vi "ModuFPGA.vi"() -> ()   [LabVIEW 2012]
uses:
  <vilib>/Platform/TimedLoop/XDataNode/timing_clust.ctl
  <vilib>/Platform/TimedLoop/XDataNode/nitl_modes.ctl
  <vilib>/Platform/TimedLoop/XDataNode/wakeup.ctl
  <vilib>/rvi/DataTransferAndStorage/Container/Common/niFpgaContainerMetaDataKey.ctl
  <vilib>/rvi/DataTransferAndStorage/Container/Common/niFpgaContainerState.ctl
  <vilib>/rvi/DataTransferAndStorage/Container/Common/niFpgaDataTypeControl.ctl
  <vilib>/rvi/DataTransferAndStorage/Container/Common/niFpgaContainerImplementationControl.ctl
  <vilib>/rvi/DataTransferAndStorage/Container/Common/niFpgaContainerArbitrationOptionsControl.ctl
  <vilib>/rvi/DataTransferAndStorage/Container/Common/niFpgaTransferTypeControl.ctl
  <vilib>/rvi/DataTransferAndStorage/Container/Common/niFpgaContainerInitializationParameters.ctl
  <vilib>/rvi/Memory/Memory_Types/niFpgaMemoryInterfaceConfiguration.ctl
  <vilib>/rvi/FIFO/Fifo_Types/niFpgaFifoControlLogicControl.ctl
  <vilib>/rvi/eio/common/nirviEmuTemplateMethod_errors.vi
  <vilib>/rvi/FIFO/Fifo_Resource/nirvififoEmulationSetSize.vi
  <vilib>/rvi/DataTransferAndStorage/Container/Common/niFpgaContainerGetUniqueNameForEmu.vi
  <vilib>/rvi/Emulation/niFpgaSctlEmulationRegisterWithScheduler.vi
  <vilib>/rvi/Emulation/niFpgaSctlEmulationScheduler.vi
  <vilib>/rvi/DataTransferAndStorage/Container/Common/niFpgaContainerSetEmuInfo.vi
  <vilib>/rvi/eio/common/nirviEmuReportErrorAndStop.vi
  <vilib>/rvi/Emulation/niFpgaSctlEmulationFifoFullMgr.vi
  <vilib>/rvi/errors/niFpgaSetErrorForExecOnDevCompSimple.vi
  <vilib>/rvi/Memory/Memory_Emulation/niFpgaMemoryEmulationCacheClearOnFirstRun.vi
  <vilib>/rvi/Memory/Memory_Emulation/nirvimemoryEmulationManagerCache_MakeExclusive.vi
  <vilib>/rvi/Memory/Memory_Emulation/niFpgaMemoryEmulationValidateCache.vi
  <vilib>/rvi/Memory/Memory_Emulation/nirvimemoryEmulationManagerCache_ReleaseExclusive.vi
  <vilib>/rvi/Memory/Memory_Emulation/nirvimemoryEmulationManagerCache_InsertValue.vi
  <vilib>/Utility/error.llb/Clear Errors.vi
  <vilib>/rvi/Memory/Memory_Emulation/nirvimemoryEmulationManagerCache_GetValue.vi
  <vilib>/rvi/Emulation/niFpgaSctlEmulationResourceMgr.vi
  <vilib>/eio/EIONode/EIONode.xnode
  <vilib>/Platform/TimedLoop/XDataNode/XDataNode.xnode
  <vilib>/rvi/DataTransferAndStorage/Container/XNode/niFpgaContainer.xnode
  <vilib>/rvi/FIFO/Fifo_Resource/nirvififoEmulationClear.vi
  <vilib>/rvi/LocalResourceManager/LocalResourceManager.xnode
  <vilib>/rvi/FIFO/Fifo_Resource/nirvififoEmulationRead.vi
  <vilib>/rvi/Memory/Memory_Emulation/nirvimemoryEmulation.vi
  <vilib>/rvi/FIFO/Fifo_Resource/nirvififoEmulationWrite.vi
  <vilib>/Platform/TimedLoop/XDataNode/XDNodeRunTimeDep.lvlib
panel:
  out "Total number of pulses sent ch 0":u64
  out "Total number of pulses sent ch 1":u64
  out "Total number of pulses sent ch 2":u64
  out "Total number of pulses sent ch 3":u64
  out "Total number of pulses sent ch 4":u64
  out "Total number of pulses sent ch 5":u64
  out "Total number of pulses sent ch 6":u64
  out "Total number of pulses sent ch 7":u64
  out "IO Module\\ADC Error A":bool
  out "IO Module\\ADC Error B":bool
  out "IO Module\\Pll Unlocked":bool
  in  "Record Size only data":u32=95
  out "DMA FIFO Timed Out?":bool
  in  "circular buffer length":u32=1000
  in  "location":i16(ring) items=["Purdue", "NIKHEF", "Zurich", "???"]
  in  "Trigger 0":i16=4000
  in  "Trigger 1":i16=4000
  in  "Trigger 2":i16=4000
  in  "Trigger 3":i16=4000
  in  "Trigger 4":i16=4000
  in  "Trigger 5":i16=4000
  in  "Trigger 6":i16=4000
  in  "Trigger 7":i16=4000
  in  "# of pretrigger":u32=20
  in  "initial value":u64
  in  "channel 0 on/off":bool
  in  "channel 2 on/off":bool
  in  "channel 1 on/off":bool
  in  "channel 3 on/off":bool
  in  "channel 4 on/off":bool
  in  "channel 5 on/off":bool
  in  "channel 6 on/off":bool
  in  "channel 7 on/off":bool
  in  "Testpulse duration (20 ns ticks)":u32=1
  in  "Testpulse Separation (20 ns ticks)":u32=500
  in  "Testpulse Time Delay (20 ns ticks)":u32=15
  in  "Testpulser On/Off":bool
  out "Init Done":bool
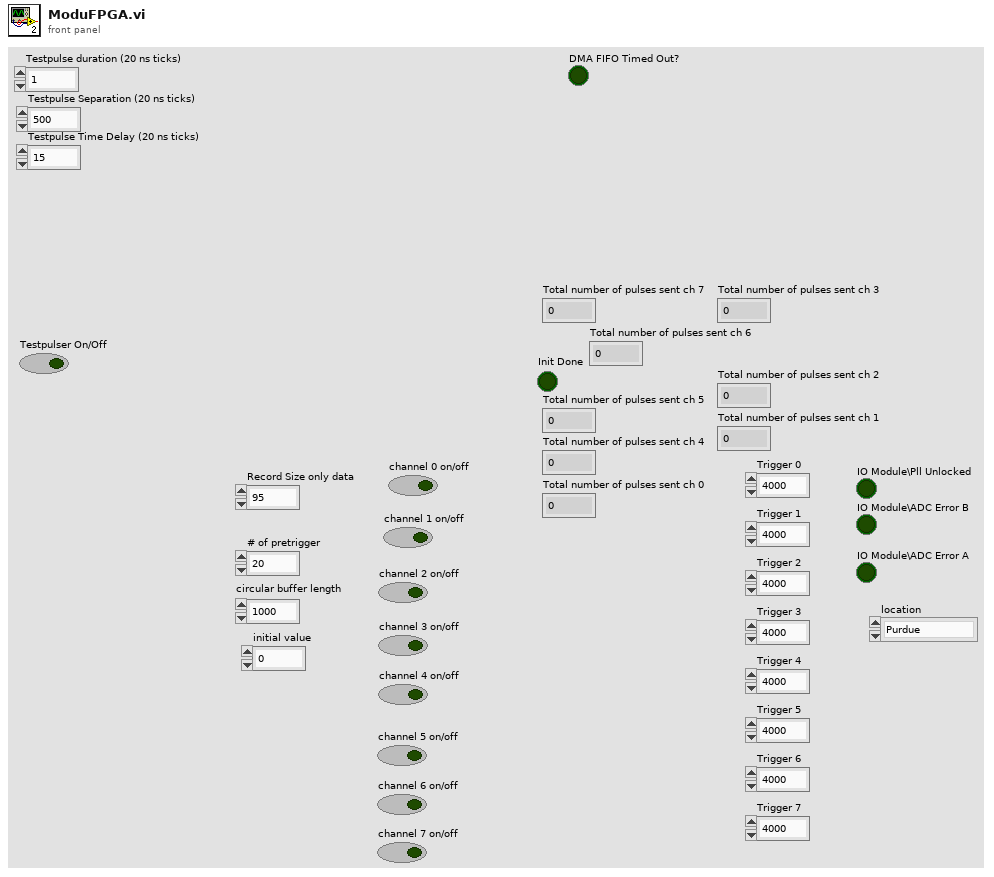
[diagram p1: front panel]
types:
  T1 = typedef "XDNodeRunTimeDep.lvlib/timing_clust.ctl" = cluster{"Expected End [f-1]":u64, "Actual End [f-1]":u64, "Finished Late? [f-1]":bool, "Expected End [i-1]":u64, "Actual End [i-1]":u64, "Finished Late? [i-1]":bool, "Expected Start [i]":u64, "Actual Start [i]":u64, "Expected Start [f]":u64, "Actual Start [f]":u64, "Source Name":string, "Structure Name":string, "Period":i64, "Deadline":i64, "Offset":i64, "Start":i64, "Priority":i32, "Timeout":i32, "Mode":T2, "Wakeup Reason":T3, "Error":errorcluster, "Source Type":string, "Secondary Source Type":string, "Global End Time":u64, "Global Start Time":u64, "Frame Duration":u64, "Iteration Duration":u64, "Assigned CPU":i32, "I/O Scan Engine Mode":u32}
  T2 = typedef "XDNodeRunTimeDep.lvlib/nitl_modes.ctl" = enum32{"No Change", "Process missed periods, maintain original phase", "Discard missed periods, maintain original phase", "Process missed periods, ignore original phase", "Discard missed periods, ignore original phase"}
  T3 = typedef "XDNodeRunTimeDep.lvlib/wakeup.ctl" = enum32{"Normal", "Aborted", "Asynchronous wakeup", "Timing source error", "Timed loop error", "Timeout"}
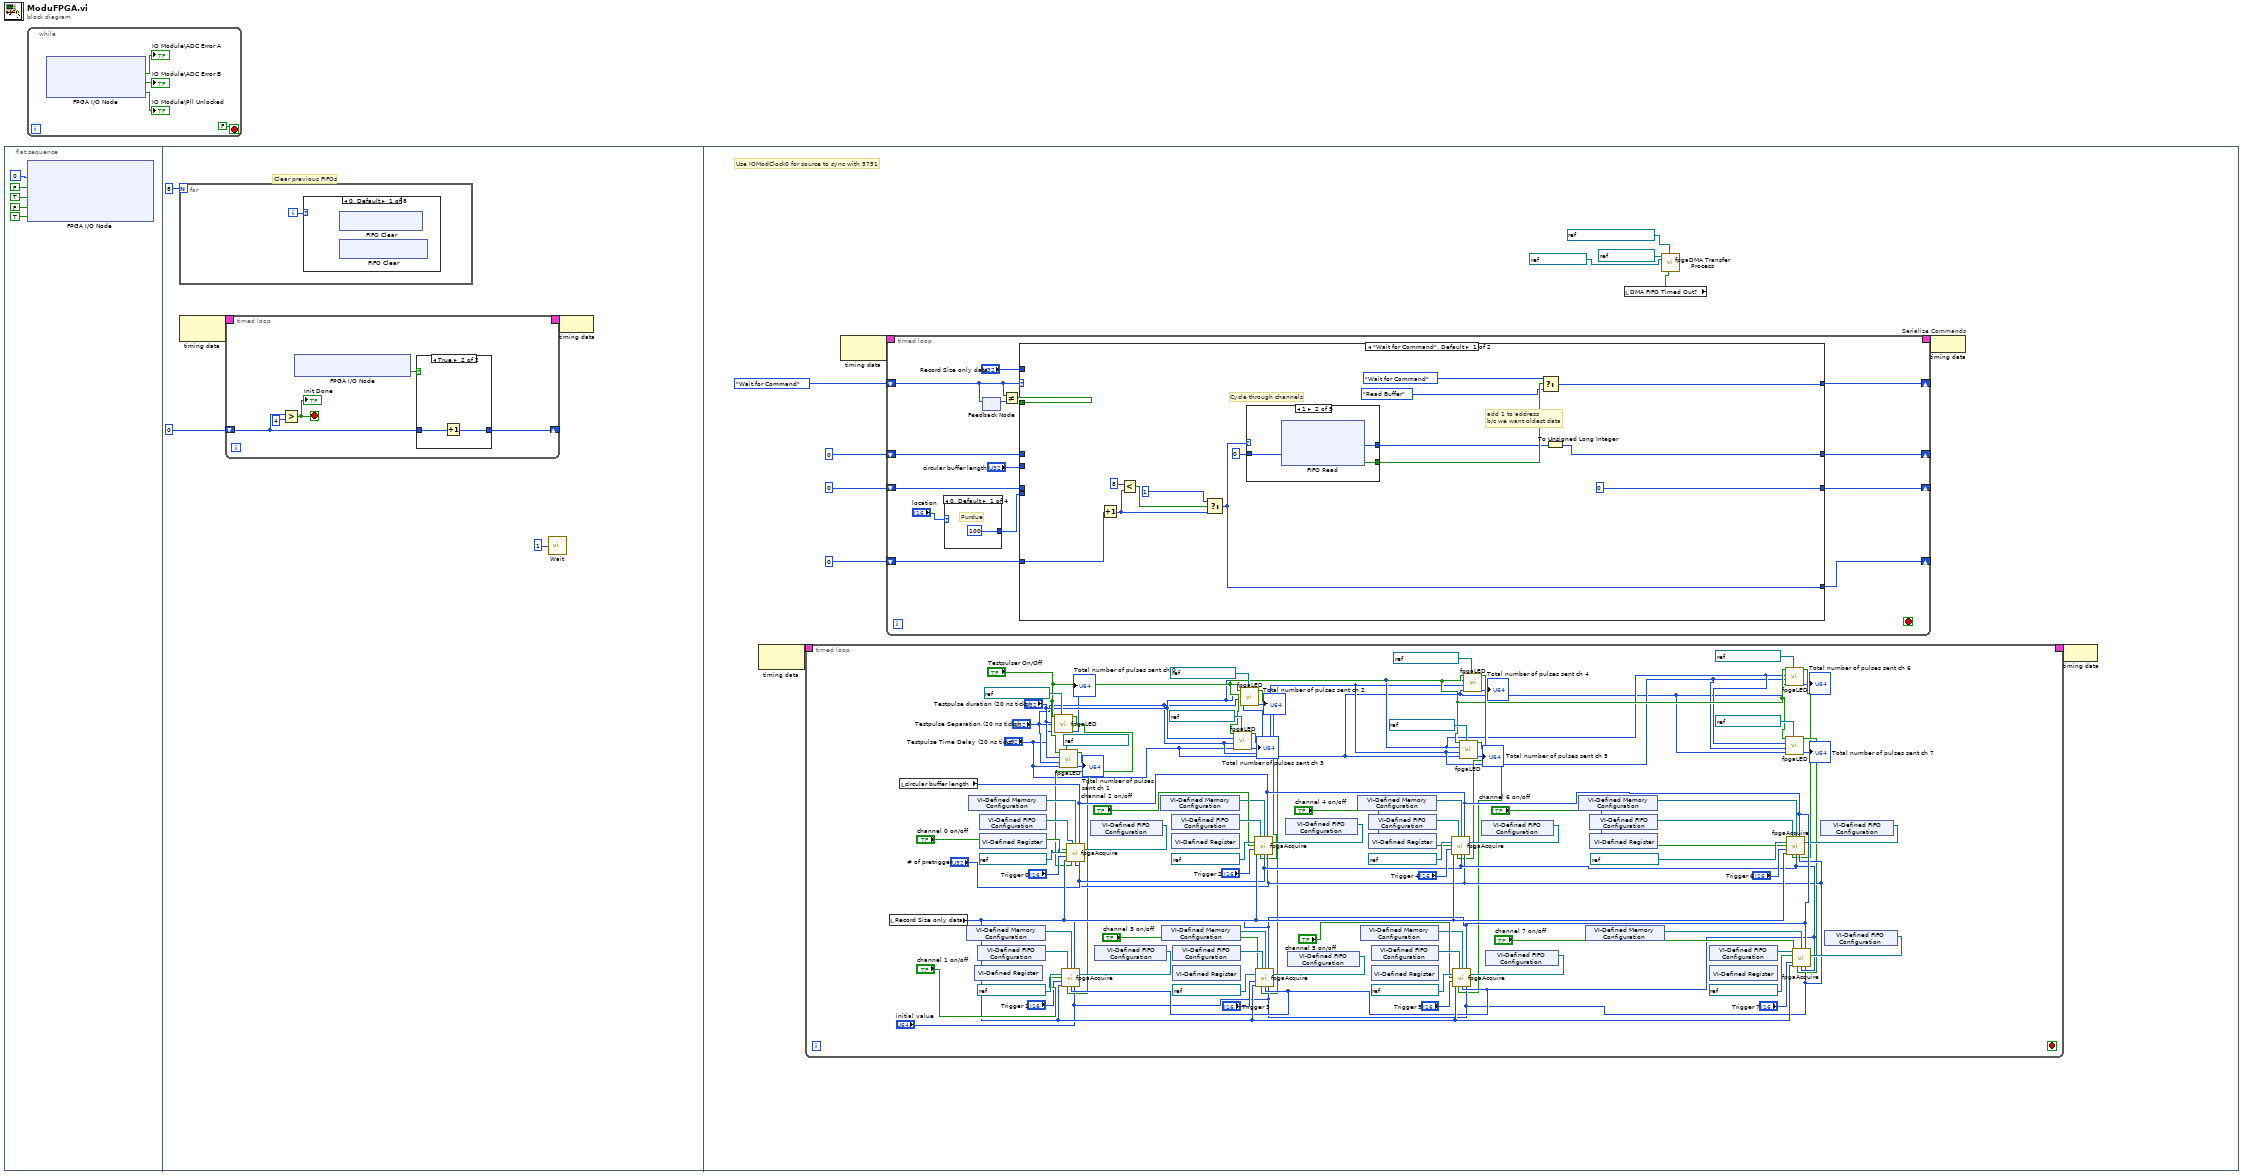
[diagram p0: block diagram]
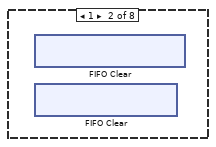
[diagram p2: hidden frame]
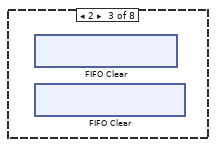
[diagram p3: hidden frame]
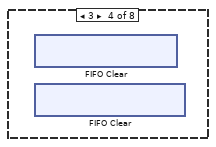
[diagram p4: hidden frame]
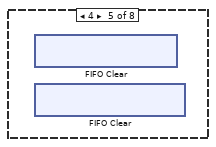
[diagram p5: hidden frame]
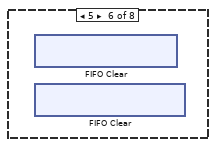
[diagram p6: hidden frame]
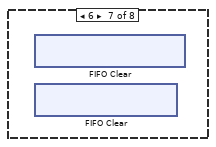
[diagram p7: hidden frame]
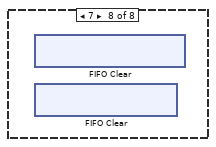
[diagram p8: hidden frame]
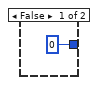
[diagram p9: hidden frame]
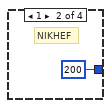
[diagram p10: hidden frame]
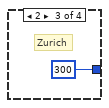
[diagram p11: hidden frame]
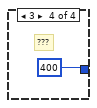
[diagram p12: hidden frame]
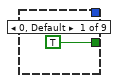
[diagram p13: hidden frame]
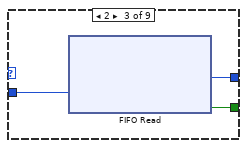
[diagram p14: hidden frame]
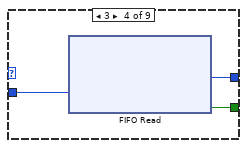
[diagram p15: hidden frame]
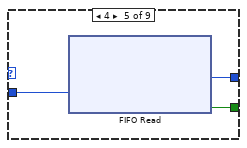
[diagram p16: hidden frame]
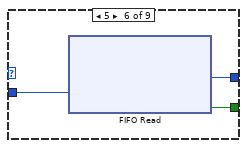
[diagram p17: hidden frame]
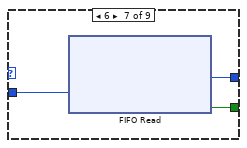
[diagram p18: hidden frame]
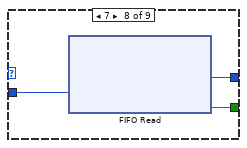
[diagram p19: hidden frame]
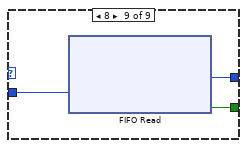
[diagram p20: hidden frame]
diagram:
  n1 = flat-sequence {
    frame #0 {
      n2 = xnode "FPGA I/O Node"("IO Module\\Sample Clock Select"=u8 0 ("IO Module\\Sample Clock Select"), "IO Module\\Force Initialization"=FALSE ("IO Module\\Force Initialization"), "IO Module\\Force Initialization"=TRUE ("IO Module\\Force Initialization"), "IO Module\\Force Initialization"=FALSE ("IO Module\\Force Initialization"), "IO Module\\Digital Output Enable"=TRUE ("IO Module\\Digital Output Enable")) -> ()  [unwired: 5 in, 5 out]
    }
    frame #1 {
      # "Clear previous FIFOs"
      n3 = for {
        N: 8 -> [_]
        i -> [w11]
        n4 = case shown="0, Default" w11 {
          frame 0, Default {
            n5 = xnode ("FIFO Clear")() -> ()  [unwired: 1 in, 1 out]
            n6 = xnode ("FIFO Clear")() -> ()  [unwired: 1 in, 1 out]
          }
          frame 1 {
            n7 = xnode ("FIFO Clear")() -> ()  [unwired: 1 in, 1 out]
            n8 = xnode ("FIFO Clear")() -> ()  [unwired: 1 in, 1 out]
          }
          frame 2 {
            n9 = xnode ("FIFO Clear")() -> ()  [unwired: 1 in, 1 out]
            n10 = xnode ("FIFO Clear")() -> ()  [unwired: 1 in, 1 out]
          }
          frame 3 {
            n11 = xnode ("FIFO Clear")() -> ()  [unwired: 1 in, 1 out]
            n12 = xnode ("FIFO Clear")() -> ()  [unwired: 1 in, 1 out]
          }
          frame 4 {
            n13 = xnode ("FIFO Clear")() -> ()  [unwired: 1 in, 1 out]
            n14 = xnode ("FIFO Clear")() -> ()  [unwired: 1 in, 1 out]
          }
          frame 5 {
            n15 = xnode ("FIFO Clear")() -> ()  [unwired: 1 in, 1 out]
            n16 = xnode ("FIFO Clear")() -> ()  [unwired: 1 in, 1 out]
          }
          frame 6 {
            n17 = xnode ("FIFO Clear")() -> ()  [unwired: 1 in, 1 out]
            n18 = xnode ("FIFO Clear")() -> ()  [unwired: 1 in, 1 out]
          }
          frame 7 {
            n19 = xnode ("FIFO Clear")() -> ()  [unwired: 1 in, 1 out]
            n20 = xnode ("FIFO Clear")() -> ()  [unwired: 1 in, 1 out]
          }
        }
      }
      n21 = node-c288() -> (w10:T1)  [unwired: 1 in]
      n22 = timed-loop {
        shift-right: [w15] -> _
        shift-left: u16 0 -> [w14]
        timing: w10 -> [_]
        timing-out: [_] -> w9
        stop <- w12 stop-if-true
        n23 = Greater?(x=w14, y=u16 4) -> (0:w12:bool)
        "Init Done" <- w12
        n24 = xnode "FPGA I/O Node"() -> ("IO Module\\Initialization Done"=w16:bool)  [unwired: 1 in, 1 out]
        n25 = case shown="True" w16 {
          tunnel: [u16 0 w19] -> w15
          tunnel: w14 -> [_ w18]
          frame False {
          }
          frame True {
            n26 = Increment(x=w18) -> (x+1=w19:u16)
          }
        }
      }
      n27 = call "Wait"("Count(mSec)"=u32 1) -> ()  [unwired: 1 out]
      n28 = node-c288(w9) -> ()
    }
    frame #2 {
      # "Use IOModClock0 for source to sync with 5751"
      n29 = node-c288() -> (w29:T1)  [unwired: 1 in]
      n30 = timed-loop {
        timing: w29 -> [_]
        timing-out: [_] -> w28
        stop <- _ stop-if-true
        n31 = local read "Record Size only data"() -> (w91:u32)
        n32 = local read "circular buffer length"() -> (w66:u32)
        n33 = xnode "VI-Defined Memory Configuration"() -> ("Memory Out"=w67:refnum<k21>)
        n34 = xnode "VI-Defined Memory Configuration"() -> ("Memory Out"=w74:refnum<k21>)
        n35 = xnode "VI-Defined Register"() -> ()  [unwired: 1 out]
        n36 = xnode "VI-Defined FIFO Configuration"() -> ("FIFO Out"=w115:refnum<k21>)
        n37 = xnode "VI-Defined FIFO Configuration"() -> ("FIFO Out"=w92:refnum<k21>)
        n38 = xnode "VI-Defined Register"() -> ()  [unwired: 1 out]
        n39 = call "fpgaLED.vi"("FPGA I/O In"=refnum<k21> "IO Module\\D0 0", "Testpulse Time Delay (20 ns ticks)"="Testpulse Time Delay (20 ns ticks)", "Testpulse Separation (20 ns ticks)"="Testpulse Separation (20 ns ticks)", "Testpulse duration (20 ns ticks)"="Testpulse duration (20 ns ticks)", "Testpulser On/Off"="Testpulser On/Off") -> ("Total number of pulses sent"=→"Total number of pulses sent ch 0":u64, "Is Test Pulse?"=w48:bool)  [unwired: 5 in]
        n40 = call "fpgaLED.vi"("FPGA I/O In"=refnum<k21> "IO Module\\D0 1", "Testpulse Time Delay (20 ns ticks)"="Testpulse Time Delay (20 ns ticks)", "Testpulse Separation (20 ns ticks)"="Testpulse Separation (20 ns ticks)", "Testpulse duration (20 ns ticks)"="Testpulse duration (20 ns ticks)", "Testpulser On/Off"="Testpulser On/Off") -> ("Total number of pulses sent"=→"Total number of pulses sent ch 1":u64, "Is Test Pulse?"=w49:bool)  [unwired: 5 in]
        n41 = xnode "VI-Defined FIFO Configuration"() -> ("FIFO Out"=w64:refnum<k21>)
        n42 = call "fpgaAcquire.vi"("Command FIFO"=w92, "Circular Buffer Mem"=w74, "circular buffer length"=w66, "FPGA I/O In"=refnum<k21> "IO Module\\AI A0", "Timing FIFO"=w64, "channel on/off"="channel 0 on/off", "Trigger"="Trigger 0", "Samples to Acquire"=w91, "Is Test Pulse?"=w48, "# of pretrigger"="# of pretrigger", "timing"="initial value") -> ()  [unwired: 5 in]
        n43 = xnode "VI-Defined FIFO Configuration"() -> ("FIFO Out"=w65:refnum<k21>)
        n44 = call "fpgaAcquire.vi"("Command FIFO"=w115, "Circular Buffer Mem"=w67, "circular buffer length"=w66, "FPGA I/O In"=refnum<k21> "IO Module\\AI A1", "Timing FIFO"=w65, "channel on/off"="channel 1 on/off", "Trigger"="Trigger 1", "Samples to Acquire"=w91, "Is Test Pulse?"=w49, "# of pretrigger"="# of pretrigger", "timing"="initial value") -> ()  [unwired: 5 in]
        n45 = xnode "VI-Defined Memory Configuration"() -> ("Memory Out"=w73:refnum<k21>)
        n46 = xnode "VI-Defined Memory Configuration"() -> ("Memory Out"=w68:refnum<k21>)
        n47 = xnode "VI-Defined FIFO Configuration"() -> ("FIFO Out"=w113:refnum<k21>)
        n48 = xnode "VI-Defined Register"() -> ()  [unwired: 1 out]
        n49 = xnode "VI-Defined FIFO Configuration"() -> ("FIFO Out"=w114:refnum<k21>)
        n50 = xnode "VI-Defined Register"() -> ()  [unwired: 1 out]
        n51 = call "fpgaLED.vi"("FPGA I/O In"=refnum<k21> "IO Module\\D0 3", "Testpulse Time Delay (20 ns ticks)"="Testpulse Time Delay (20 ns ticks)", "Testpulse Separation (20 ns ticks)"="Testpulse Separation (20 ns ticks)", "Testpulse duration (20 ns ticks)"="Testpulse duration (20 ns ticks)", "Testpulser On/Off"="Testpulser On/Off") -> ("Total number of pulses sent"=→"Total number of pulses sent ch 3":u64, "Is Test Pulse?"=w51:bool)  [unwired: 5 in]
        n52 = call "fpgaLED.vi"("FPGA I/O In"=refnum<k21> "IO Module\\D0 2", "Testpulse Time Delay (20 ns ticks)"="Testpulse Time Delay (20 ns ticks)", "Testpulse Separation (20 ns ticks)"="Testpulse Separation (20 ns ticks)", "Testpulse duration (20 ns ticks)"="Testpulse duration (20 ns ticks)", "Testpulser On/Off"="Testpulser On/Off") -> ("Total number of pulses sent"=→"Total number of pulses sent ch 2":u64, "Is Test Pulse?"=w50:bool)  [unwired: 5 in]
        n53 = xnode "VI-Defined FIFO Configuration"() -> ("FIFO Out"=w63:refnum<k21>)
        n54 = call "fpgaAcquire.vi"("Command FIFO"=w113, "Circular Buffer Mem"=w73, "circular buffer length"=w66, "FPGA I/O In"=refnum<k21> "IO Module\\AI A2", "Timing FIFO"=w63, "channel on/off"="channel 2 on/off", "Trigger"="Trigger 2", "Samples to Acquire"=w91, "Is Test Pulse?"=w50, "# of pretrigger"="# of pretrigger", "timing"="initial value") -> ()  [unwired: 5 in]
        n55 = xnode "VI-Defined FIFO Configuration"() -> ("FIFO Out"=w62:refnum<k21>)
        n56 = call "fpgaAcquire.vi"("Command FIFO"=w114, "Circular Buffer Mem"=w68, "circular buffer length"=w66, "FPGA I/O In"=refnum<k21> "IO Module\\AI A3", "Timing FIFO"=w62, "channel on/off"="channel 3 on/off", "Trigger"="Trigger 3", "Samples to Acquire"=w91, "Is Test Pulse?"=w51, "# of pretrigger"="# of pretrigger", "timing"="initial value") -> ()  [unwired: 5 in]
        n57 = xnode "VI-Defined Memory Configuration"() -> ("Memory Out"=w72:refnum<k21>)
        n58 = xnode "VI-Defined Memory Configuration"() -> ("Memory Out"=w69:refnum<k21>)
        n59 = xnode "VI-Defined Register"() -> ()  [unwired: 1 out]
        n60 = xnode "VI-Defined FIFO Configuration"() -> ("FIFO Out"=w109:refnum<k21>)
        n61 = xnode "VI-Defined FIFO Configuration"() -> ("FIFO Out"=w110:refnum<k21>)
        n62 = xnode "VI-Defined Register"() -> ()  [unwired: 1 out]
        n63 = call "fpgaLED.vi"("FPGA I/O In"=refnum<k21> "IO Module\\D0 5", "Testpulse Time Delay (20 ns ticks)"="Testpulse Time Delay (20 ns ticks)", "Testpulse Separation (20 ns ticks)"="Testpulse Separation (20 ns ticks)", "Testpulse duration (20 ns ticks)"="Testpulse duration (20 ns ticks)", "Testpulser On/Off"="Testpulser On/Off") -> ("Total number of pulses sent"=→"Total number of pulses sent ch 5":u64, "Is Test Pulse?"=w53:bool)  [unwired: 5 in]
        n64 = call "fpgaLED.vi"("FPGA I/O In"=refnum<k21> "IO Module\\D0 4", "Testpulse Time Delay (20 ns ticks)"="Testpulse Time Delay (20 ns ticks)", "Testpulse Separation (20 ns ticks)"="Testpulse Separation (20 ns ticks)", "Testpulse duration (20 ns ticks)"="Testpulse duration (20 ns ticks)", "Testpulser On/Off"="Testpulser On/Off") -> ("Total number of pulses sent"=→"Total number of pulses sent ch 4":u64, "Is Test Pulse?"=w52:bool)  [unwired: 5 in]
        n65 = xnode "VI-Defined FIFO Configuration"() -> ("FIFO Out"=w58:refnum<k21>)
        n66 = call "fpgaAcquire.vi"("Command FIFO"=w109, "Circular Buffer Mem"=w72, "circular buffer length"=w66, "FPGA I/O In"=refnum<k21> "IO Module\\AI A4", "Timing FIFO"=w58, "channel on/off"="channel 4 on/off", "Trigger"="Trigger 4", "Samples to Acquire"=w91, "Is Test Pulse?"=w52, "# of pretrigger"="# of pretrigger", "timing"="initial value") -> ()  [unwired: 5 in]
        n67 = xnode "VI-Defined FIFO Configuration"() -> ("FIFO Out"=w61:refnum<k21>)
        n68 = call "fpgaAcquire.vi"("Command FIFO"=w110, "Circular Buffer Mem"=w69, "circular buffer length"=w66, "FPGA I/O In"=refnum<k21> "IO Module\\AI A5", "Timing FIFO"=w61, "channel on/off"="channel 5 on/off", "Trigger"="Trigger 5", "Samples to Acquire"=w91, "Is Test Pulse?"=w53, "# of pretrigger"="# of pretrigger", "timing"="initial value") -> ()  [unwired: 5 in]
        n69 = xnode "VI-Defined Memory Configuration"() -> ("Memory Out"=w71:refnum<k21>)
        n70 = xnode "VI-Defined Memory Configuration"() -> ("Memory Out"=w70:refnum<k21>)
        n71 = xnode "VI-Defined FIFO Configuration"() -> ("FIFO Out"=w112:refnum<k21>)
        n72 = xnode "VI-Defined Register"() -> ()  [unwired: 1 out]
        n73 = xnode "VI-Defined FIFO Configuration"() -> ("FIFO Out"=w111:refnum<k21>)
        n74 = xnode "VI-Defined Register"() -> ()  [unwired: 1 out]
        n75 = call "fpgaLED.vi"("FPGA I/O In"=refnum<k21> "IO Module\\D0 6", "Testpulse Time Delay (20 ns ticks)"="Testpulse Time Delay (20 ns ticks)", "Testpulse Separation (20 ns ticks)"="Testpulse Separation (20 ns ticks)", "Testpulse duration (20 ns ticks)"="Testpulse duration (20 ns ticks)", "Testpulser On/Off"="Testpulser On/Off") -> ("Total number of pulses sent"=→"Total number of pulses sent ch 6":u64, "Is Test Pulse?"=w54:bool)  [unwired: 5 in]
        n76 = call "fpgaLED.vi"("FPGA I/O In"=refnum<k21> "IO Module\\D0 7", "Testpulse Time Delay (20 ns ticks)"="Testpulse Time Delay (20 ns ticks)", "Testpulse Separation (20 ns ticks)"="Testpulse Separation (20 ns ticks)", "Testpulse duration (20 ns ticks)"="Testpulse duration (20 ns ticks)", "Testpulser On/Off"="Testpulser On/Off") -> ("Total number of pulses sent"=→"Total number of pulses sent ch 7":u64, "Is Test Pulse?"=w55:bool)  [unwired: 5 in]
        n77 = xnode "VI-Defined FIFO Configuration"() -> ("FIFO Out"=w59:refnum<k21>)
        n78 = call "fpgaAcquire.vi"("Command FIFO"=w112, "Circular Buffer Mem"=w71, "circular buffer length"=w66, "FPGA I/O In"=refnum<k21> "IO Module\\AI A6", "Timing FIFO"=w59, "channel on/off"="channel 6 on/off", "Trigger"="Trigger 6", "Samples to Acquire"=w91, "Is Test Pulse?"=w54, "# of pretrigger"="# of pretrigger", "timing"="initial value") -> ()  [unwired: 5 in]
        n79 = xnode "VI-Defined FIFO Configuration"() -> ("FIFO Out"=w60:refnum<k21>)
        n80 = call "fpgaAcquire.vi"("Command FIFO"=w111, "Circular Buffer Mem"=w70, "circular buffer length"=w66, "FPGA I/O In"=refnum<k21> "IO Module\\AI A7", "Timing FIFO"=w60, "channel on/off"="channel 7 on/off", "Trigger"="Trigger 7", "Samples to Acquire"=w91, "Is Test Pulse?"=w55, "# of pretrigger"="# of pretrigger", "timing"="initial value") -> ()  [unwired: 5 in]
      }
      n81 = node-c288() -> (w31:T1)  [unwired: 1 in]
      n82 = timed-loop "Serialize Commands" {
        timing: w31 -> [_]
        timing-out: [_] -> w30
        shift-right: [w896] -> _
        shift-left: enum16{"Wait for Command", "Read Buffer"}."Wait for Command" -> [w894]
        shift-right: [w900] -> _
        shift-left: u32 0 ("Element") -> [w899]
        shift-right: [w898] -> _
        shift-left: u8 0 ("t") -> [w897]
        shift-right: [w891] -> _
        shift-left: u64 0 ("Element") -> [w890]
        stop <- _ stop-if-true
        n83 = case shown="0, Default" "location" {
          tunnel: [i16 100 i16 200 i16 300 i16 400] -> w888
          frame 0, Default {
            # "Purdue"
          }
          frame 1 {
            # "NIKHEF"
          }
          frame 2 {
            # "Zurich"
          }
          frame 3 {
            # "???"
          }
        }
        n84 = feedback-in #1(w894) -> ()
        n85 = feedback #1() -> (w895:enum16{"Wait for Command", "Read Buffer"})  [unwired: 1 in]
        n86 = Not Equal?(x=w894, y=w895) -> (x != y?=w892:bool)
        n87 = case shown="\"Wait for Command\", Default" w894 {
          tunnel: "Record Size only data" -> [_ w954]
          tunnel: [w908 w964] -> w898
          tunnel: w897 -> [w910 w964]
          tunnel: [w911 w949] -> w900
          tunnel: w899 -> [_ w963]
          tunnel: [w914 w965] -> w896
          tunnel: "circular buffer length" -> [_ w962]
          tunnel: w892 -> [_ w956]
          tunnel: [u64 0 ("Element") w951] -> w891
          tunnel: w890 -> [_ w950]
          tunnel: w888 -> [_ w945]
          frame "Wait for Command", Default {
            # "add 1 to address\nb/c we want oldest data"
            # "Cycle through channels"
            n88 = Increment(x=w910) -> (x+1=w909:u8)
            n89 = Less?(x=u8 8, y=w909) -> (x < y?=w918:bool)
            n90 = Select(t=u8 1, s=w918, f=w909) -> (s? t:f=w908:u8)
            n91 = case shown="1" w908 {
              tunnel: [TRUE ("Timed Out?") w923 w924 w927 w930 w933 w936 w939 w942] -> w915
              tunnel: 0 ("Timeout") -> [_ w922 w926 w929 w932 w935 w938 w941 w944]
              tunnel: [_ w921 w925 w928 w931 w934 w937 w940 w943] -> w907
              frame 0, Default {
              }
              frame 1 {
                n92 = xnode ("FIFO Read")("Timeout"=w922) -> ("Element"=w921:i16, "Timed Out?"=w923:bool)  [unwired: 1 in, 1 out]
              }
              frame 2 {
                n93 = xnode ("FIFO Read")("Timeout"=w926) -> ("Element"=w925:i16, "Timed Out?"=w924:bool)  [unwired: 1 in, 1 out]
              }
              frame 3 {
                n94 = xnode ("FIFO Read")("Timeout"=w929) -> ("Element"=w928:i16, "Timed Out?"=w927:bool)  [unwired: 1 in, 1 out]
              }
              frame 4 {
                n95 = xnode ("FIFO Read")("Timeout"=w932) -> ("Element"=w931:i16, "Timed Out?"=w930:bool)  [unwired: 1 in, 1 out]
              }
              frame 5 {
                n96 = xnode ("FIFO Read")("Timeout"=w935) -> ("Element"=w934:i16, "Timed Out?"=w933:bool)  [unwired: 1 in, 1 out]
              }
              frame 6 {
                n97 = xnode ("FIFO Read")("Timeout"=w938) -> ("Element"=w937:i16, "Timed Out?"=w936:bool)  [unwired: 1 in, 1 out]
              }
              frame 7 {
                n98 = xnode ("FIFO Read")("Timeout"=w941) -> ("Element"=w940:i16, "Timed Out?"=w939:bool)  [unwired: 1 in, 1 out]
              }
              frame 8 {
                n99 = xnode ("FIFO Read")("Timeout"=w944) -> ("Element"=w943:i16, "Timed Out?"=w942:bool)  [unwired: 1 in, 1 out]
              }
            }
            n100 = Select(t=enum16{"Wait for Command", "Read Buffer"}."Wait for Command", s=w915, f=enum16{"Wait for Command", "Read Buffer"}."Read Buffer") -> (s? t:f=w914:enum16{"Wait for Command", "Read Buffer"})
            n101 = To Unsigned Long Integer(number=w907) -> (unsigned 32bit integer=w911:u32)
          }
          frame "Read Buffer" {
            # "the first 5 entries are reserved for channel and 4 timing info"
            # "add timeouts"
            n102 = feedback #2() -> (w948:bool)  [unwired: 1 in]
            n103 = Add(x=w954, y=u32 5) -> (x+y=w952:u32)
            n104 = call "fpgaCount Up.vi"("Reset?"=w956, "goal"=w952) -> ("Count Met"=w958:bool, "count"=w955:u32)  [unwired: 8 in]
            n105 = case shown="0, Default" w955 {
              tunnel: w964 -> [_ w974 w981 _ _ _ w1020]
              tunnel: w963 -> [_ w978 w983 w1004 w1010 w1016 w1026]
              tunnel: w962 -> [_ _ _ _ _ _ w1025]
              tunnel: [i16 0 ("Data") w975 w985 w1002 w1008 w1014 w1021] -> w957
              tunnel: w948 -> [_ _ _ _ _ _ w1023]
              tunnel: [u64 0 ("Element") _ w982 w1005 w1011 w1017 _] -> w951
              tunnel: w950 -> [_ _ _ w1005 w1011 w1017 _]
              tunnel: [u32 0 ("Element") w978 w983 w1004 w1010 w1016 _] -> w949
              tunnel: [FALSE FALSE FALSE FALSE FALSE TRUE FALSE] -> w947
              tunnel: w945 -> [_ w970 _ _ _ _ _]
              frame 0, Default {
              }
              frame 1 {
                w976 = u16 0 items=["Header Information", "Particle Pulse", "Test Pulse"] ("Pulse Type")
                n106 = Decrement(x=w974) -> (x-1=w973:u8)
                n107 = To Word Integer(number=w973) -> (16bit integer=w972:i16)
                n108 = Add(x=w970, y=w972) -> (x+y=w971:i16)
                n109 = call "fpgaBit Manipulation.vi"("Pulse Type"=w976, "Integer to be written"=w971) -> ("Integer Written"=w975:i16)  [unwired: 2 in]
              }
              frame 2 {
                # "reads out the lsb of the timing information"
                n110 = case shown="Default" w981 {
                  tunnel: [_ w986 w988 w990 w992 w994 w996 w998 w1000] -> w982
                  frame Default {
                  }
                  frame 1 {
                    n111 = xnode ("FIFO Read")("Timeout"=0) -> ("Element"=w986:u64)  [unwired: 1 in, 2 out]
                  }
                  frame 2 {
                    n112 = xnode ("FIFO Read")("Timeout"=0) -> ("Element"=w988:u64)  [unwired: 1 in, 2 out]
                  }
                  frame 3 {
                    n113 = xnode ("FIFO Read")("Timeout"=0) -> ("Element"=w990:u64)  [unwired: 1 in, 2 out]
                  }
                  frame 4 {
                    n114 = xnode ("FIFO Read")("Timeout"=0) -> ("Element"=w992:u64)  [unwired: 1 in, 2 out]
                  }
                  frame 5 {
                    n115 = xnode ("FIFO Read")("Timeout"=0) -> ("Element"=w994:u64)  [unwired: 1 in, 2 out]
                  }
                  frame 6 {
                    n116 = xnode ("FIFO Read")("Timeout"=0) -> ("Element"=w996:u64)  [unwired: 1 in, 2 out]
                  }
                  frame 7 {
                    n117 = xnode ("FIFO Read")("Timeout"=0) -> ("Element"=w998:u64)  [unwired: 1 in, 2 out]
                  }
                  frame 8 {
                    n118 = xnode ("FIFO Read")("Timeout"=0) -> ("Element"=w1000:u64)  [unwired: 1 in, 2 out]
                  }
                }
                n119 = Split Number(x=w982) -> (hi(x)=w980:u32)  [unwired: 1 out]
                n120 = Split Number(x=w980) -> (hi(x)=w979:u16)  [unwired: 1 out]
                n121 = To Word Integer(number=w979) -> (16bit integer=w985:i16)
              }
              frame 3 {
                n122 = Split Number(x=w1005) -> (hi(x)=w1007:u32)  [unwired: 1 out]
                n123 = Split Number(x=w1007) -> (lo(x)=w1006:u16)  [unwired: 1 out]
                n124 = To Word Integer(number=w1006) -> (16bit integer=w1002:i16)
              }
              frame 4 {
                n125 = Split Number(x=w1011) -> (lo(x)=w1013:u32)  [unwired: 1 out]
                n126 = Split Number(x=w1013) -> (hi(x)=w1012:u16)  [unwired: 1 out]
                n127 = To Word Integer(number=w1012) -> (16bit integer=w1008:i16)
              }
              frame 5 {
                n128 = Split Number(x=w1017) -> (lo(x)=w1019:u32)  [unwired: 1 out]
                n129 = Split Number(x=w1019) -> (lo(x)=w1018:u16)  [unwired: 1 out]
                n130 = To Word Integer(number=w1018) -> (16bit integer=w1014:i16)
              }
              frame 6.. {
                n131 = call "fpgaCircular Buffer Address.vi"("Reset?"=w1023, "Starting Address"=w1026, "circular buffer length"=w1025) -> ("Address"=w1024:u32)  [unwired: 8 in]
                n132 = case shown="1" w1020 {
                  tunnel: w1024 -> [_ w1029 w1031 w1033 w1035 w1037 w1039 w1041 w1043]
                  tunnel: [i16 0 w1028 w1030 w1032 w1034 w1036 w1038 w1040 w1042] -> w1021
                  frame Default {
                    # "Error"
                  }
                  frame 1 {
                    n133 = xnode ("Memory Read")("Address"=w1029) -> ("Data"=w1028:i16)  [unwired: 1 in, 1 out]
                  }
                  frame 2 {
                    n134 = xnode ("Memory Read")("Address"=w1031) -> ("Data"=w1030:i16)  [unwired: 1 in, 1 out]
                  }
                  frame 3 {
                    n135 = xnode ("Memory Read")("Address"=w1033) -> ("Data"=w1032:i16)  [unwired: 1 in, 1 out]
                  }
                  frame 4 {
                    n136 = xnode ("Memory Read")("Address"=w1035) -> ("Data"=w1034:i16)  [unwired: 1 in, 1 out]
                  }
                  frame 5 {
                    n137 = xnode ("Memory Read")("Address"=w1037) -> ("Data"=w1036:i16)  [unwired: 1 in, 1 out]
                  }
                  frame 6 {
                    n138 = xnode ("Memory Read")("Address"=w1039) -> ("Data"=w1038:i16)  [unwired: 1 in, 1 out]
                  }
                  frame 7 {
                    n139 = xnode ("Memory Read")("Address"=w1041) -> ("Data"=w1040:i16)  [unwired: 1 in, 1 out]
                  }
                  frame 8 {
                    n140 = xnode ("Memory Read")("Address"=w1043) -> ("Data"=w1042:i16)  [unwired: 1 in, 1 out]
                  }
                }
              }
            }
            n141 = feedback-in #2(w947) -> ()
            n142 = xnode ("FIFO Read")("Element"=w957, "Timeout"=0) -> ("Timed Out?"=→"DMA FIFO Timed Out?":bool)  [unwired: 1 in, 1 out]
            n143 = Select(t=enum16{"Wait for Command", "Read Buffer"}."Wait for Command", s=w958, f=enum16{"Wait for Command", "Read Buffer"}."Read Buffer") -> (s? t:f=w965:enum16{"Wait for Command", "Read Buffer"})
          }
        }
      }
      n144 = local read "DMA FIFO Timed Out?"() -> (w32:bool)
      n145 = call "fpgaDMA Transfer Process.vi"("DMA Write Timed Out?"=w32, "Clock Domain"=refnum<k21> "40 MHz Onboard Clock", "Local"=refnum<k21> "To DMA FIFO", "DMA"=refnum<k21> "To Host FIFO") -> ()  [unwired: 8 in]
      n146 = node-c288(w30) -> ()
      n147 = node-c288(w28) -> ()
    }
  }
  n148 = while {
    stop <- FALSE stop-if-true
    n149 = xnode "FPGA I/O Node"() -> ("IO Module\\ADC Error A"=→"IO Module\\ADC Error A":bool, "IO Module\\ADC Error B"=→"IO Module\\ADC Error B":bool, "IO Module\\Pll Unlocked"=→"IO Module\\Pll Unlocked":bool)  [unwired: 3 in, 3 out]
  }
